vi "28[6]-Remote Control[RCMD].vi"(8 "error in (no error)":errorcluster, 11 "S2F41":T2) -> (0 "error out":errorcluster, 2 "Timeout?":bool, 3 "S2F42":T1)   [LabVIEW 2020, in "SECS Scenarios.lvlib" / "Scenarios Class.lvclass"]
uses:
  Scenarios Class.lvclass
  SECS Communication/S2 Message Class/S2F41.ctl
  SECS Communication/S2 Message Class/S2F42.ctl
  28[6]-Remote Control[RCMD].ctl
  SECS Communication/S2 Message Class/S2 Message Class.lvclass
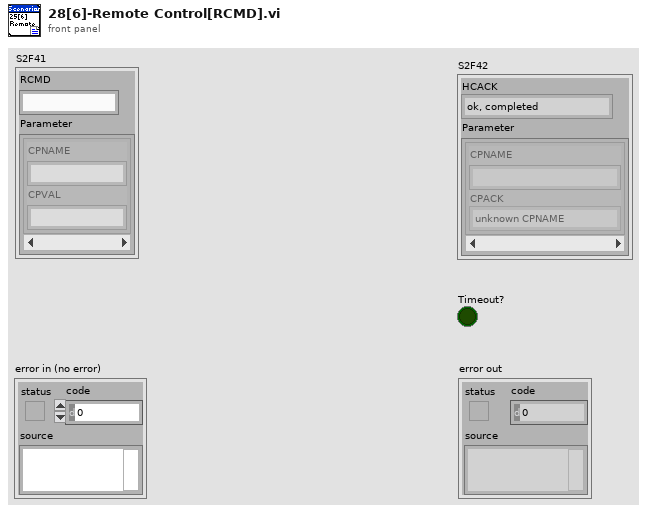
[diagram p1: front panel]
types:
  T1 = typedef "SECS Communication.lvlib/S2 Message Class.lvclass/S2F42.ctl" = cluster{"HCACK":enum8{"ok, completed", "invalid command", "cannot do now", "parameter error", "initiated for asynchronous completion", "rejected, already in desired condition", "invalid object"}, "Parameter ":cluster{"CPNAME":string, "CPACK":enum8{"unknown CPNAME", "illegal value for CPVAL", "illegal format for CPVAL"}}[]}
  T2 = typedef "SECS Communication.lvlib/S2 Message Class.lvclass/S2F41.ctl" = cluster{"RCMD":string, "Parameter":cluster{"CPNAME":string, "CPVAL":string}[]}
  T3 = typedef "SECS Scenarios.lvlib/Scenarios Class.lvclass/28[6]-Remote Control[RCMD].ctl" = cluster{"S2F41":T2, "Reply Notifier":refnum<notifier>}
  T4 = typedef "SECS Scenarios.lvlib/Scenarios Class.lvclass/Broadcast Refnum.ctl" = cluster{"13-EnableDisable Alarm":refnum<user-event>, "15-Process Program Request":refnum<user-event>, "16-Process Program Send":refnum<user-event>, "17-Deleting a Process Program by Host":refnum<user-event>, "18-Host Requests Equipment Process Program Directory":refnum<user-event>, "19-Equipment Process Program Uploading":refnum<user-event>, "20[1]-Process Program Downloading":refnum<user-event>, "20[2]-Process Program Downloading":refnum<user-event>, "22-Host Sends Information to Equipment":refnum<user-event>, "26-Host Requests to Enter OFF-Line":refnum<user-event>, "27-Host Requests to Enter On-Line":refnum<user-event>, "28[1]-Remote Control[PP-SELECT]":refnum<user-event>, "28[2]-Remote Control[START]":refnum<user-event>, "28[3]-Remote Control[STOP]":refnum<user-event>, "28[4]-Remote Control[LOCAL]":refnum<user-event>, "28[5]-Remote Control[REMOTE]":refnum<user-event>, "28[6]-Remote Control[RCMD]":refnum<user-event>, "30-Host Requests Equipment to Set Time":refnum<user-event>, "31-Host Requests Time Value from Equipment":refnum<user-event>, "32[1]-Trace Data Collection":refnum<user-event>, "32[2]-Trace Data Collection":refnum<user-event>}
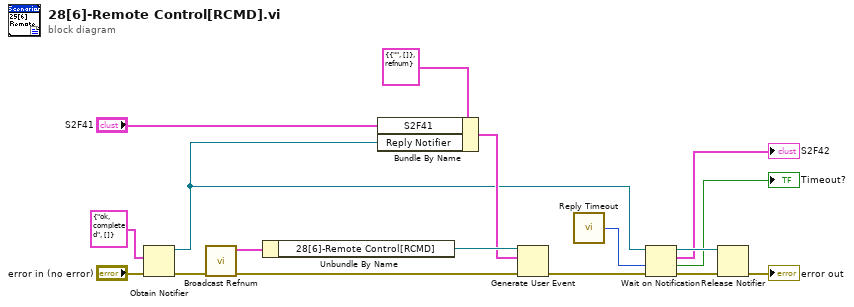
[diagram p0: block diagram]
diagram:
  n1 = Obtain Notifier(notification data type=T1 {"HCACK"=enum."ok, completed", "Parameter "=[]} ("S2F42"), error in (no error)="error in (no error)") -> (notifier out=w2:refnum<notifier>, error out=w16:errorcluster)  [unwired: 2 in, 1 out]
  n2 = call "Broadcast Refnum.vi"("error in"=w16) -> ("error out"=w15:errorcluster, "Broadcast Refnum"=w17:T4)  [unwired: 9 in]
  n3 = Unbundle By Name(w17) -> ("28[6]-Remote Control[RCMD]"=w14:refnum<user-event>)
  n4 = Bundle By Name(cluster=T3 {"S2F41"={"RCMD"="", "Parameter"=[]}, "Reply Notifier"=refnum} ("28[6]-Remote Control[RCMD]"), "S2F41"="S2F41", "Reply Notifier"=w2) -> (w6:T3)
  n5 = Generate User Event(user event=w14, event data cluster=w6, error in=w15) -> (error out=w13:errorcluster)  [unwired: 1 in, 1 out]
  n6 = call "Reply Timeout.vi"() -> ("Reply Timeout"=w12:i32)
  n7 = Wait on Notification(notifier=w2, timeout in ms (-1)=w12, error in (no error)=w13) -> (notifier out=w11:refnum<notifier>, notification=→"S2F42":T1, timed out?=→"Timeout?":bool, error out=w10:errorcluster)  [unwired: 1 in]
  n8 = Release Notifier(notifier=w11, error in (no error)=w10) -> (error out=→"error out":errorcluster)  [unwired: 1 in, 2 out]
